vi "hCalRT2013.vi"(0 "FPGA VI Reference In":refnum<k20>, 5 "cancelbutton":refnum<vi>, 7 "state":refnum<vi>, 9 "Acquired Samples":refnum<vi>, 11 "error in":errorcluster) -> (3 "Fehler":bool, 4 "FPGA VI Reference Out":refnum<k20>, 6 "Ref":i16[][](array[numeric]), 8 "Meas":i16[][](array[numeric]), 15 "error out":errorcluster)   [LabVIEW 2014]
uses:
  <vilib>/rvi/errors/niLvFpgaAdjustHostInterfaceError.vi
  <vilib>/Utility/error.llb/Error Cluster From Error Code.vi
  <vilib>/rvi/interface/nirviReadWriteControl/nirviReadWriteControl.xnode
  FPGA Bitfiles/W7XBolo2017_FPGATarget_fmain2014_9xlV3GyHFfo.lvbitx
  f_main_2014.vi
  NiFpgaLv.dll
panel:
  out "error out 2":errorcluster
  out "ScanID":u32
  out "error in 2":errorcluster
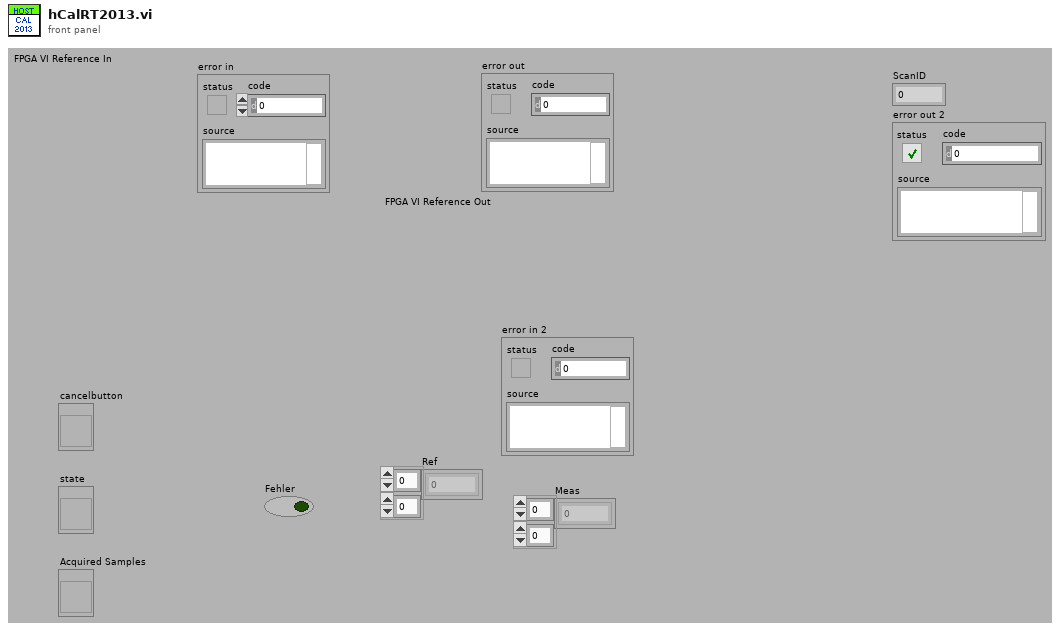
[diagram p1: front panel]
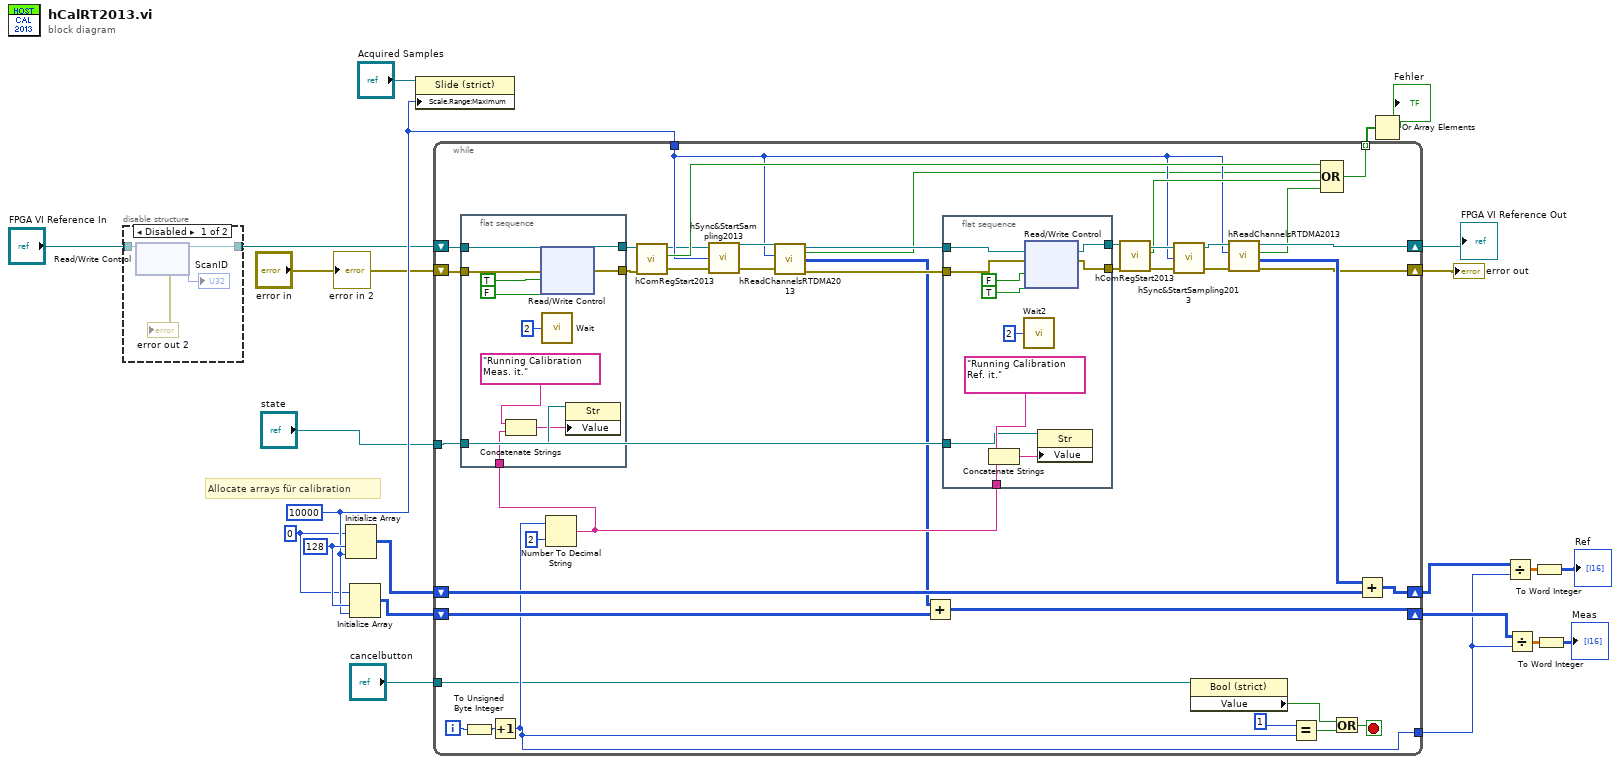
[diagram p0: block diagram]
diagram:
  w19 = 10000
  w20 = 128 ("dimension size")
  w16 = 0 ("element")
  # "Allocate arrays für calibration"
  n1 = disable-structure shown="Disabled" {
    disable-tunnel: "FPGA VI Reference In" -> [w24 w27]
    disable-tunnel: [w23 w27] -> w1
    frame Disabled {
      n2 = xnode "Read/Write Control"("FPGA VI Reference In"=w24) -> ("FPGA VI Reference Out"=w23:refnum<k20>, "error out"=→"error out 2":errorcluster, "ScanID"=→"ScanID":u32)  [unwired: 1 in]
    }
    frame Enabled {
    }
  }
  n3 = Initialize Array(w16, w20, w19) -> (w18:i32[][])
  n4 = Initialize Array(w16, w20, w19) -> (w17:i32[][])
  n5 = property on="Property Node" class="Slide (strict)"(reference="Acquired Samples", "Scale.Range:Maximum"=w19) -> ()  [unwired: 1 in, 2 out]
  n6 = while {
    shift-right: [w41] -> w3
    shift-left: w1 -> [w65]
    shift-right: [w38] -> w14
    shift-left: "error in" -> [w64]
    tunnel: w19 -> [w32]
    shift-right: [w53] -> w8
    shift-left: w18 -> [w54]
    shift-right: [w52] -> w7
    shift-left: w17 -> [w55]
    tunnel: [w48] -> w6
    tunnel: [w45] -> w22 mode=indexing
    tunnel: "cancelbutton" -> [w44]
    tunnel: "state" -> [w43]
    i -> [w61]
    stop <- w60 stop-if-true
    n7 = flat-sequence {
      tunnel: [w87] -> w68
      tunnel: [w86] -> w29
      tunnel: w65 -> [w85]
      tunnel: w64 -> [w84]
      tunnel: w58 -> [w82]
      tunnel: w43 -> [w81]
      frame #0 {
        n8 = Concatenate Strings("Running Calibration Meas. it." ("state"), w82) -> (w80:string)
        n9 = xnode "Read/Write Control"("FPGA VI Reference In"=w85, "error in"=w84, "RLY1"=TRUE ("RESET"), "RLY2"=FALSE ("RESET")) -> ("FPGA VI Reference Out"=w86:refnum<k20>, "error out"=w87:errorcluster)
        n10 = call "Wait"("Count(mSec)"=u8 2 ("Count(uSec)")) -> ()  [unwired: 1 out]
        n11 = property class="Str"(reference=w81, "Value"=w80) -> ()  [unwired: 1 in, 2 out]
      }
    }
    n12 = To Unsigned Byte Integer(number=w61) -> (unsigned 8bit integer=w57:u8)
    n13 = Increment(x=w57) -> (x+1=w48:u8)
    n14 = Number To Decimal String(number=w48, width (-)=u8 2) -> (decimal integer string=w58:string)
    n15 = call "hComRegStart2013.vi"("error in"=w68, "FPGA VI Reference In"=w29) -> ("error out"=w51:errorcluster, "Timed Out"=w47:bool, "FPGA VI Reference Out"=w28:refnum<k20>)  [unwired: 3 in]
    n16 = call "hSync&StartSampling2013.vi"("error in"=w51, "#Samples"=w32, "FPGA VI Reference In"=w28) -> ("error out"=w35:errorcluster, "FPGA VI Reference Out"=w36:refnum<k20>)  [unwired: 1 in]
    n17 = call "hReadChannelsRTDMA2013.vi"("FPGA VI Reference In"=w36, "Nsamples"=w32, "error in"=w35) -> ("FPGA VI Reference Out"=w34:refnum<k20>, "Fehler"=w31:bool, "RawArray"=w30:i16[][], "error out"=w33:errorcluster)  [unwired: 2 in]
    n18 = Add(x=w30, y=w55) -> (x+y=w52:i32[][])
    n19 = flat-sequence {
      tunnel: w34 -> [w76]
      tunnel: w33 -> [w75]
      tunnel: [w74] -> w67
      tunnel: [w73] -> w66
      tunnel: w58 -> [w70]
      tunnel: w43 -> [w69]
      frame #0 {
        n20 = Concatenate Strings("Running Calibration Ref. it." ("state"), w70) -> (w72:string)
        n21 = call "Wait2"("Count(mSec)"=u16 2 ("Count(uSec)")) -> ()  [unwired: 1 out]
        n22 = xnode "Read/Write Control"("FPGA VI Reference In"=w76, "error in"=w75, "RLY1"=FALSE ("RESET"), "RLY2"=TRUE ("RESET")) -> ("FPGA VI Reference Out"=w74:refnum<k20>, "error out"=w73:errorcluster)
        n23 = property class="Str"(reference=w69, "Value"=w72) -> ()  [unwired: 1 in, 2 out]
      }
    }
    n24 = call "hComRegStart2013.vi"("error in"=w66, "FPGA VI Reference In"=w67) -> ("error out"=w49:errorcluster, "Timed Out"=w46:bool, "FPGA VI Reference Out"=w50:refnum<k20>)  [unwired: 3 in]
    n25 = call "hSync&StartSampling2013.vi"("error in"=w49, "#Samples"=w32, "FPGA VI Reference In"=w50) -> ("error out"=w37:errorcluster, "FPGA VI Reference Out"=w42:refnum<k20>)  [unwired: 1 in]
    n26 = property class="Bool (strict)"(reference=w44) -> ("Value"=w56:bool)  [unwired: 1 in, 2 out]
    n27 = call "hReadChannelsRTDMA2013.vi"("FPGA VI Reference In"=w42, "Nsamples"=w32, "error in"=w37) -> ("FPGA VI Reference Out"=w41:refnum<k20>, "Fehler"=w39:bool, "RawArray"=w40:i16[][], "error out"=w38:errorcluster)  [unwired: 2 in]
    n28 = Equal?(x=u8 1, y=w48) -> (x = y?=w59:bool)
    n29 = Compound Arithmetic op=OR(w47, w31, w46, w39) -> (w45:bool)
    n30 = Or(x=w56, y=w59) -> (x .or. y?=w60:bool)
    n31 = Add(x=w40, y=w54) -> (x+y=w53:i32[][])
  }
  "error out" <- w14
  "FPGA VI Reference Out" <- w3
  n32 = Or Array Elements(Boolean array=w22) -> (logical OR=→"Fehler":bool)
  n33 = Divide(x=w8, y=w6) -> (x/y=w9:dbl[][])
  n34 = Divide(x=w7, y=w6) -> (x/y=w10:dbl[][])
  n35 = To Word Integer(number=w9) -> (16bit integer=→"Ref":i16[][])
  n36 = To Word Integer(number=w10) -> (16bit integer=→"Meas":i16[][])
  "error in 2" <- "error in"
